vi "LEDC SWIR 2936 Main.vi"(0 "LEDAD Port":refnum<visa-resource-name>="COM7", 2 "Unit":u16(ring) items=["nW/cm^2", "pW/cm^2"], 5 "Light Meter Port":refnum<visa-resource-name>="COM4", 7 "Intensity Desired":dbl(slide) scale=0.0..100.0, 9 "Enable LED":u8(slide) scale=0.0..31.0, 11 "error in (no error)":errorcluster, 12 "Channel":enum16{"Chn1", "Chn2"}(ring)) -> (3 "In Progress":bool, 4 "LEDAD Port out":refnum<visa-resource-name>, 6 "Light Meter Port out":refnum<visa-resource-name>, 8 "Meas Illum":dbl format="%#_4g", 14 "Done":bool, 15 "error out":errorcluster)   [LabVIEW 2010]
panel:
  # "%"
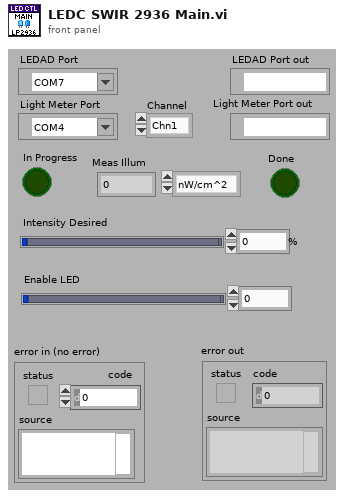
[diagram p1: front panel]
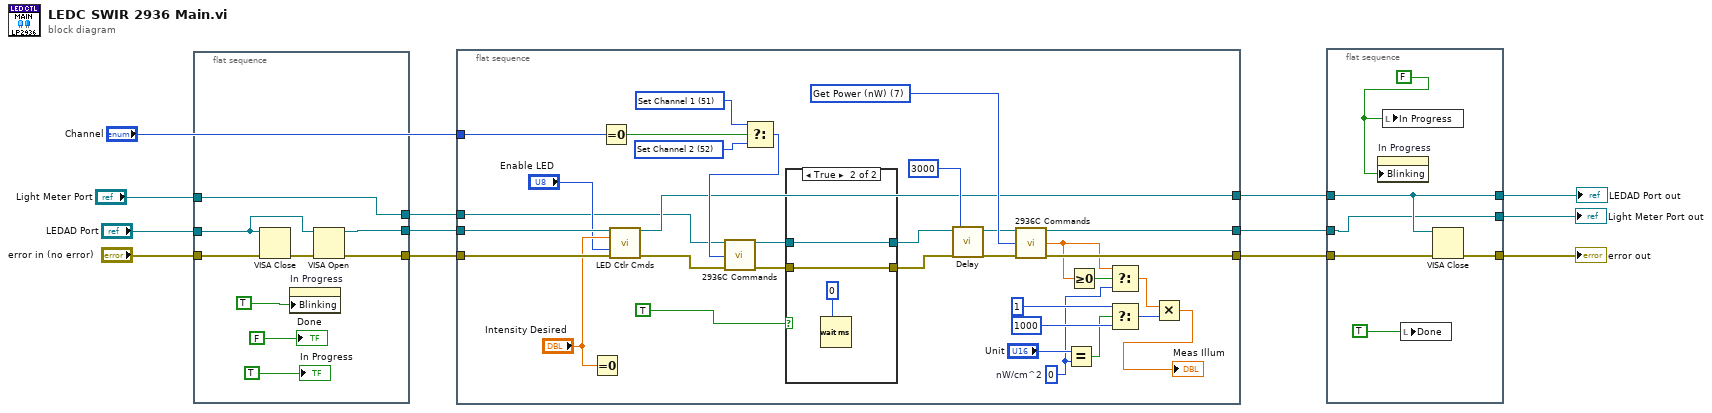
[diagram p0: block diagram]
diagram:
  n1 = flat-sequence {
    tunnel: "LEDAD Port" -> [w15]
    tunnel: [w17] -> w5
    tunnel: "error in (no error)" -> [w18]
    tunnel: [w16] -> w7
    tunnel: "Light Meter Port" -> [w14]
    tunnel: [w14] -> w6
    frame #0 {
      n2 = VISA Close(VISA resource name=w15, error in (no error)=w18) -> (error out=w19:errorcluster)
      n3 = property on="In Progress" class="Bool (strict)"("Blinking"=TRUE) -> ()  [unwired: 2 in, 2 out]
      n4 = VISA Open(error in (no error)=w19, VISA resource name=w15) -> (VISA resource name=w16:refnum<visa-resource-name>, error out=w17:errorcluster)  [unwired: 3 in]
      "Done" <- FALSE
      "In Progress" <- TRUE
    }
  }
  n5 = flat-sequence {
    tunnel: w5 -> [w41]
    tunnel: w7 -> [w42]
    tunnel: w6 -> [w24]
    tunnel: [w50] -> w13
    tunnel: [w25] -> w11
    tunnel: [w49] -> w12
    tunnel: "Channel" -> [w33]
    frame #0 {
      w35 = u16 52 items=["Attenuator OFF", "Attenuator ON", "Attenuator Query", "Beep OFF", "Beep ON", "Beep Query", "Clear Status Reg", "Get Power (nW)", "Echo OFF", "Echo ON", "Echo Query", "No Filter", "Analog Filter", "Digital FIlter", "Filter Query", "Hold", "Go", "Go Query", "Backlight OFF", "Backlight Medium", "Backlight High", "Backlight Query", "Set Dsplay Screen 0", "Set Display Screen 1", "Display Screen Query", "Mode DC Continuous", "Mode DC Single", "Mode Integrate", "Identification", "Auto Range", "Auto Range Query", "Signal Range 0", "Signal Range 1", "Signal Range 2", "Signal Range 3", "Signal Range 4", "Signal Range 5", "Signal Range 6", "Signal Range Query", "Store Reference", "Units W", "Units W/cm2", "Units dBm", "Units Joules", "Units Query", "Set Wavelength", "Wavelength Querry", "Mode Pesk-to-Peak Cont.", "Mode Peak-to-Peak Sing.", "Mode Query", "Channel Querry", "Set Channel 1", "Set Channel 2"] ("Command")
      w36 = u16 51 items=["Attenuator OFF", "Attenuator ON", "Attenuator Query", "Beep OFF", "Beep ON", "Beep Query", "Clear Status Reg", "Get Power (nW)", "Echo OFF", "Echo ON", "Echo Query", "No Filter", "Analog Filter", "Digital FIlter", "Filter Query", "Hold", "Go", "Go Query", "Backlight OFF", "Backlight Medium", "Backlight High", "Backlight Query", "Set Dsplay Screen 0", "Set Display Screen 1", "Display Screen Query", "Mode DC Continuous", "Mode DC Single", "Mode Integrate", "Identification", "Auto Range", "Auto Range Query", "Signal Range 0", "Signal Range 1", "Signal Range 2", "Signal Range 3", "Signal Range 4", "Signal Range 5", "Signal Range 6", "Signal Range Query", "Store Reference", "Units W", "Units W/cm2", "Units dBm", "Units Joules", "Units Query", "Set Wavelength", "Wavelength Querry", "Mode Pesk-to-Peak Cont.", "Mode Peak-to-Peak Sing.", "Mode Query", "Channel Querry", "Set Channel 1", "Set Channel 2"] ("Command")
      w37 = u16 7 items=["Attenuator OFF", "Attenuator ON", "Attenuator Query", "Beep OFF", "Beep ON", "Beep Query", "Clear Status Reg", "Get Power (nW)", "Echo OFF", "Echo ON", "Echo Query", "No Filter", "Analog Filter", "Digital FIlter", "Filter Query", "Hold", "Go", "Go Query", "Backlight OFF", "Backlight Medium", "Backlight High", "Backlight Query", "Set Dsplay Screen 0", "Set Display Screen 1", "Display Screen Query", "Mode DC Continuous", "Mode DC Single", "Mode Integrate", "Identification", "Auto Range", "Auto Range Query", "Signal Range 0", "Signal Range 1", "Signal Range 2", "Signal Range 3", "Signal Range 4", "Signal Range 5", "Signal Range 6", "Signal Range Query", "Store Reference", "Units W", "Units W/cm2", "Units dBm", "Units Joules", "Units Query", "Set Wavelength", "Wavelength Querry", "Mode Pesk-to-Peak Cont.", "Mode Peak-to-Peak Sing.", "Mode Query", "Channel Querry", "Set Channel 1", "Set Channel 2"] ("Command")
      w44 = 0  # nW/cm^2
      n6 = Equal To 0?(x="Intensity Desired") -> ()  [unwired: 1 out]
      n7 = Equal To 0?(x=w33) -> (x = 0?=w34:bool)
      n8 = call "LED Ctlr Cmds.vi"("VISA session"=w42, "Intensity"="Intensity Desired", "Enable"="Enable LED", "error in (no error)"=w41) -> ("VISA session out"=w25:refnum<visa-resource-name>, "error out"=w29:errorcluster)  [unwired: 7 in, 3 out]
      n9 = Select(t=w36, s=w34, f=w35) -> (s? t:f=w26:u16)
      n10 = call "2936C Commands.vi"("Instrument Resource Name"=w24, "Command"=w26, "error in (no error)"=w29) -> ("VISA resource name out"=w28:refnum<visa-resource-name>, "error out"=w27:errorcluster)  [unwired: 8 in, 3 out]
      n11 = case shown="True" TRUE {
        tunnel: w27 -> [w56 w58]
        tunnel: [w56 w58] -> w30
        tunnel: [w55 w57] -> w23
        tunnel: w28 -> [w55 w57]
        frame False {
        }
        frame True {
          n12 = Wait (ms)(milliseconds to wait=0) -> ()  [unwired: 1 out]
        }
      }
      n13 = call "Delay.vi"("error in (no error)"=w30, "Delay"=3000) -> ("error out"=w32:errorcluster)  [unwired: 17 in]
      n14 = call "2936C Commands.vi"("Instrument Resource Name"=w23, "Command"=w37, "error in (no error)"=w32) -> ("VISA resource name out"=w50:refnum<visa-resource-name>, "LM Response"=w45:dbl, "error out"=w49:errorcluster)  [unwired: 8 in, 2 out]
      n15 = Equal?(x="Unit", y=w44) -> (x = y?=w52:bool)
      n16 = Greater Or Equal To 0?(x=w45) -> (x >= 0?=w46:bool)
      n17 = Select(t=w45, s=w46, f=w44) -> (s? t:f=w43:dbl)
      n18 = Select(t=1, s=w52, f=1000) -> (s? t:f=w51:i32)
      n19 = Multiply(x=w43, y=w51) -> (x*y=→"Meas Illum":dbl)
    }
  }
  n20 = flat-sequence {
    tunnel: w13 -> [w62]
    tunnel: w12 -> [w60]
    tunnel: [w63] -> w8
    tunnel: w11 -> [w63]
    tunnel: [w62] -> w9
    tunnel: [w61] -> w10
    frame #0 {
      w65 = FALSE
      n21 = property on="In Progress" class="Bool (strict)"("Blinking"=w65) -> ()  [unwired: 2 in, 2 out]
      n22 = local write "In Progress"(w65) -> ()
      n23 = local write "Done"(TRUE) -> ()
      n24 = VISA Close(VISA resource name=w63, error in (no error)=w60) -> (error out=w61:errorcluster)
    }
  }
  "LEDAD Port out" <- w8
  "Light Meter Port out" <- w9
  "error out" <- w10
